vi "GCMPlugin_CreateInputEvents.vi"(8 "error in (no error)":errorcluster) -> (0 "error out":errorcluster, 2 "EventsIn":T1)   [LabVIEW 2014, in "GCMPlugin.lvclass"]
uses:
  GCMPlugin/GCMPlugin.lvclass
  GCMPlugin_EventsIn.ctl
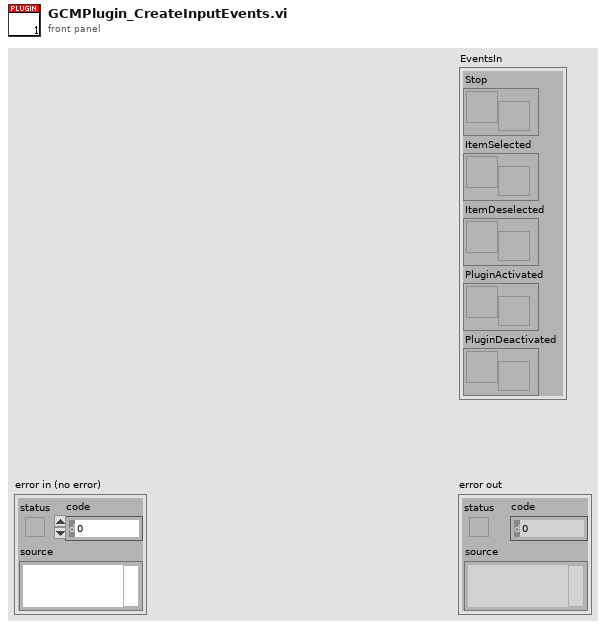
[diagram p1: front panel]
types:
  T1 = typedef "GCMPlugin.lvclass/GCMPlugin_EventsIn.ctl" = cluster{"Stop":refnum<user-event>, "ItemSelected":refnum<user-event>, "ItemDeselected":refnum<user-event>, "PluginActivated":refnum<user-event>, "PluginDeactivated":refnum<user-event>}
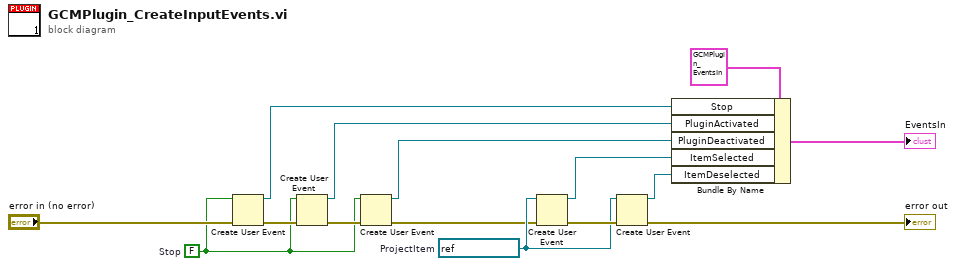
[diagram p0: block diagram]
diagram:
  w8 = refnum<vi> refnum  # ProjectItem
  w1 = FALSE  # Stop
  n1 = Create User Event(user event datatype=w1, error in="error in (no error)") -> (user event=w10:refnum<user-event>, error out=w4:errorcluster)
  n2 = Create User Event(user event datatype=w1, error in=w4) -> (user event=w6:refnum<user-event>, error out=w5:errorcluster)
  n3 = Create User Event(user event datatype=w1, error in=w5) -> (user event=w2:refnum<user-event>, error out=w3:errorcluster)
  n4 = Create User Event(user event datatype=w8, error in=w3) -> (user event=w11:refnum<user-event>, error out=w9:errorcluster)
  n5 = Create User Event(user event datatype=w8, error in=w9) -> (user event=w7:refnum<user-event>, error out=→"error out":errorcluster)
  n6 = Bundle By Name(cluster=T1 {"Stop"=refnum, "ItemSelected"=refnum, "ItemDeselected"=refnum, "PluginActivated"=refnum, "PluginDeactivated"=refnum} ("EventsIn"), "Stop"=w10, "PluginActivated"=w6, "PluginDeactivated"=w2, "ItemSelected"=w11, "ItemDeselected"=w7) -> (→"EventsIn":T1)
